vi "Exo5.vi"() -> ()   [LabVIEW 2018]
panel:
  out "Valeur tank":i16
  in  "stop":bool
  in  "Débit":dbl min=0.0 max=10.0
  out "Tank 2":i16(slide) scale=0.0..1000.0
  in  "Consigne":i16 min=0 max=1000 step=10
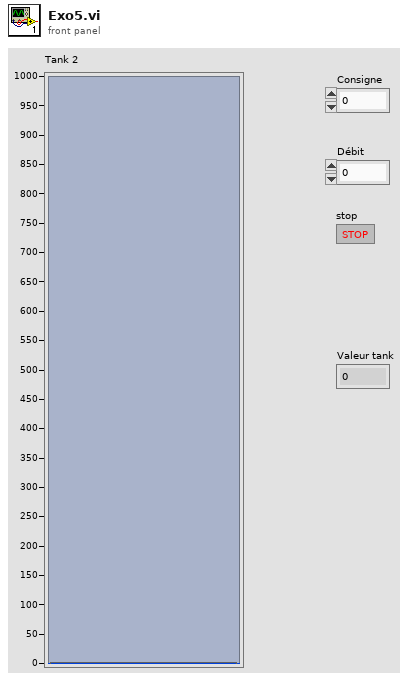
[diagram p1: front panel]
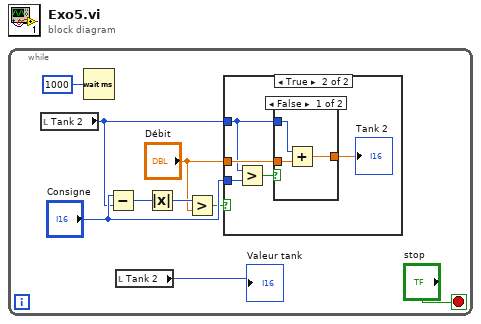
[diagram p0: block diagram]
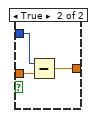
[diagram p3: hidden frame]
diagram:
  n1 = while {
    stop <- "stop" stop-if-true
    n2 = local read "Tank 2"() -> (w2:i16)
    n3 = Wait (ms)(milliseconds to wait=u32 1000) -> ()  [unwired: 1 out]
    n4 = Subtract(x="Consigne", y=w2) -> (x-y=w7:i16)
    n5 = local read "Tank 2"() -> (→"Valeur tank":i16)
    n6 = Absolute Value(x=w7) -> (abs(x)=w4:i16)
    n7 = Greater?(x=w4, y="Débit") -> (0:w5:bool)
    n8 = case shown="True" w5 {
      tunnel: "Consigne" -> [_ w12]
      tunnel: "Débit" -> [_ w11]
      tunnel: w2 -> [_ w10]
      frame False {
      }
      frame True {
        n9 = Greater?(x=w10, y=w12) -> (0:w14:bool)
        n10 = case shown="False" w14 {
          tunnel: [w15 w20] -> w13
          tunnel: w10 -> [w17 w19]
          tunnel: w11 -> [w16 w18]
          frame False {
            n11 = Add(x=w17, y=w16) -> (x+y=w15:dbl)
          }
          frame True {
            n12 = Subtract(x=w19, y=w18) -> (x-y=w20:dbl)
          }
        }
        "Tank 2" <- w13
      }
    }
  }
